vi "FP_Calibrate_reward.vi"() -> ()   [LabVIEW 2018]
uses:
  <vilib>/Instr/_visa.llb/VISA Flush IO Buffer Mask.ctl
  <vilib>/Utility/miscctls.llb/LVPointTypeDef.ctl
  Tracker.lvlib
panel:
  in  "O4 volume to dispense, µl":dbl=1.0 caption="Dispense, µl" min=0.0 max=10000.0 format="%#.3f"
  in  "O4 time to dispense, s":dbl=1.0 caption="Dispense, s" min=0.0 max=100.0 format="%.3g"
  in  "O4 Dispence, s":bool
  in  "O4 Dispence, µl":bool
  in  "O3 volume to dispense, µl":dbl=1.0 caption="Dispense, µl" min=0.0 max=10000.0 format="%#.3f"
  in  "O3 time to dispense, s":dbl=1.0 caption="Dispense, s" min=0.0 max=100.0 format="%.3g"
  in  "O3 Dispence, s":bool
  in  "O3 Dispence, µl":bool
  in  "O2 volume to dispense, µl":dbl=1.0 caption="Dispense, µl" min=0.0 max=10000.0 format="%#.3f"
  in  "O2 time to dispense, s":dbl=1.0 caption="Dispense, s" min=0.0 max=100.0 format="%.3g"
  in  "O2 Dispence, s":bool
  in  "O2 Dispence, µl":bool
  in  "O1 Dispence, µl":bool
  in  "O1 Dispence, s":bool
  in  "O1 time to dispense, s":dbl=1.0 caption="Dispense, s" min=0.0 max=100.0 format="%.3g"
  in  "O1 volume to dispense, µl":dbl=1.0 caption="Dispense, µl" min=0.0 max=10000.0 format="%#.3f"
  in  "O4 disp. time, s":dbl=1.0 min=0.0 max=100.0 format="%.3g"
  in  "O4 volume, µl":dbl=1.0 caption="Meas. volume, µl" min=0.0 max=10000.0 format="%#.3f"
  out "O4 speed, µl/s":dbl=1.0 caption="Speed, µl/s" format="%.3g"
  out "O4 act. disp. time, s":dbl=1.0 caption="Act. disp. time, s" format="%.3g"
  in  "O4 Disp. by time":bool
  in  "O3 disp. time, s":dbl=1.0 min=0.0 max=100.0 format="%.3g"
  in  "O3 volume, µl":dbl=1.0 caption="Meas. volume, µl" min=0.0 max=10000.0 format="%#.3f"
  out "O3 speed, µl/s":dbl=1.0 caption="Speed, µl/s" format="%.3g"
  out "O3 act. disp. time, s":dbl=1.0 caption="Act. disp. time, s" format="%.3g"
  in  "O3 Disp. by time":bool
  in  "O2 Disp. by time":bool
  in  "O2 disp. time, s":dbl=1.0 min=0.0 max=100.0 format="%.3g"
  in  "O2 volume, µl":dbl=1.0 caption="Meas. volume, µl" min=0.0 max=10000.0 format="%#.3f"
  out "O2 speed, µl/s":dbl=1.0 caption="Speed, µl/s" format="%.3g"
  out "O2 act. disp. time, s":dbl=1.0 caption="Act. disp. time, s" format="%.3g"
  out "O1 act. disp. time, s":dbl=1.0 caption="Act. disp. time, s" format="%.3g"
  out "O1 speed, µl/s":dbl=1.0 caption="Speed, µl/s" format="%.3g"
  in  "O1 volume, µl":dbl=1.0 caption="Meas. volume, µl" min=0.0 max=10000.0 format="%#.3f"
  in  "O1 Disp. by time":bool
  in  "O1 disp. time, s":dbl=1.0 min=0.0 max=100.0 format="%.3g"
  in  "Connect to HW":bool
  out "Ready":bool=TRUE
  out "HW info":string
  in  "Target FPS":i32=80 min=1 max=100 step=1
  in  "VISA resource":refnum<visa-resource-name>="Tracker"
  out "error out":errorcluster
  out "Sync capability":u8
  in  "error in":errorcluster
  # "O1"
  # "O2"
  # "O3"
  # "O4"
  # "Calibration"
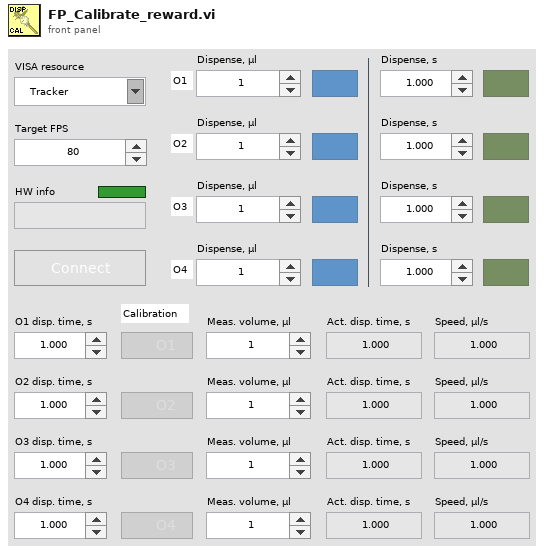
[diagram p1: front panel]
types:
  T1 = enum8{"Enabled", "Disabled", "Disabled and Grayed Out"}
  T2 = typedef "LVPointTypeDef.ctl" = cluster{"Horizontal":i16, "Vertical":i16}
  T3 = cluster{"SYNC configuration":u16, "IO 1 configuration":u16, "IO 2 configuration":u16, "IO 3 configuration":u16, "IO 4 configuration":u16, "Activate ext. RS-232":u16, "IO inversion config.":u16}
  T4 = typedef "VISA Flush IO Buffer Mask.ctl" = u16
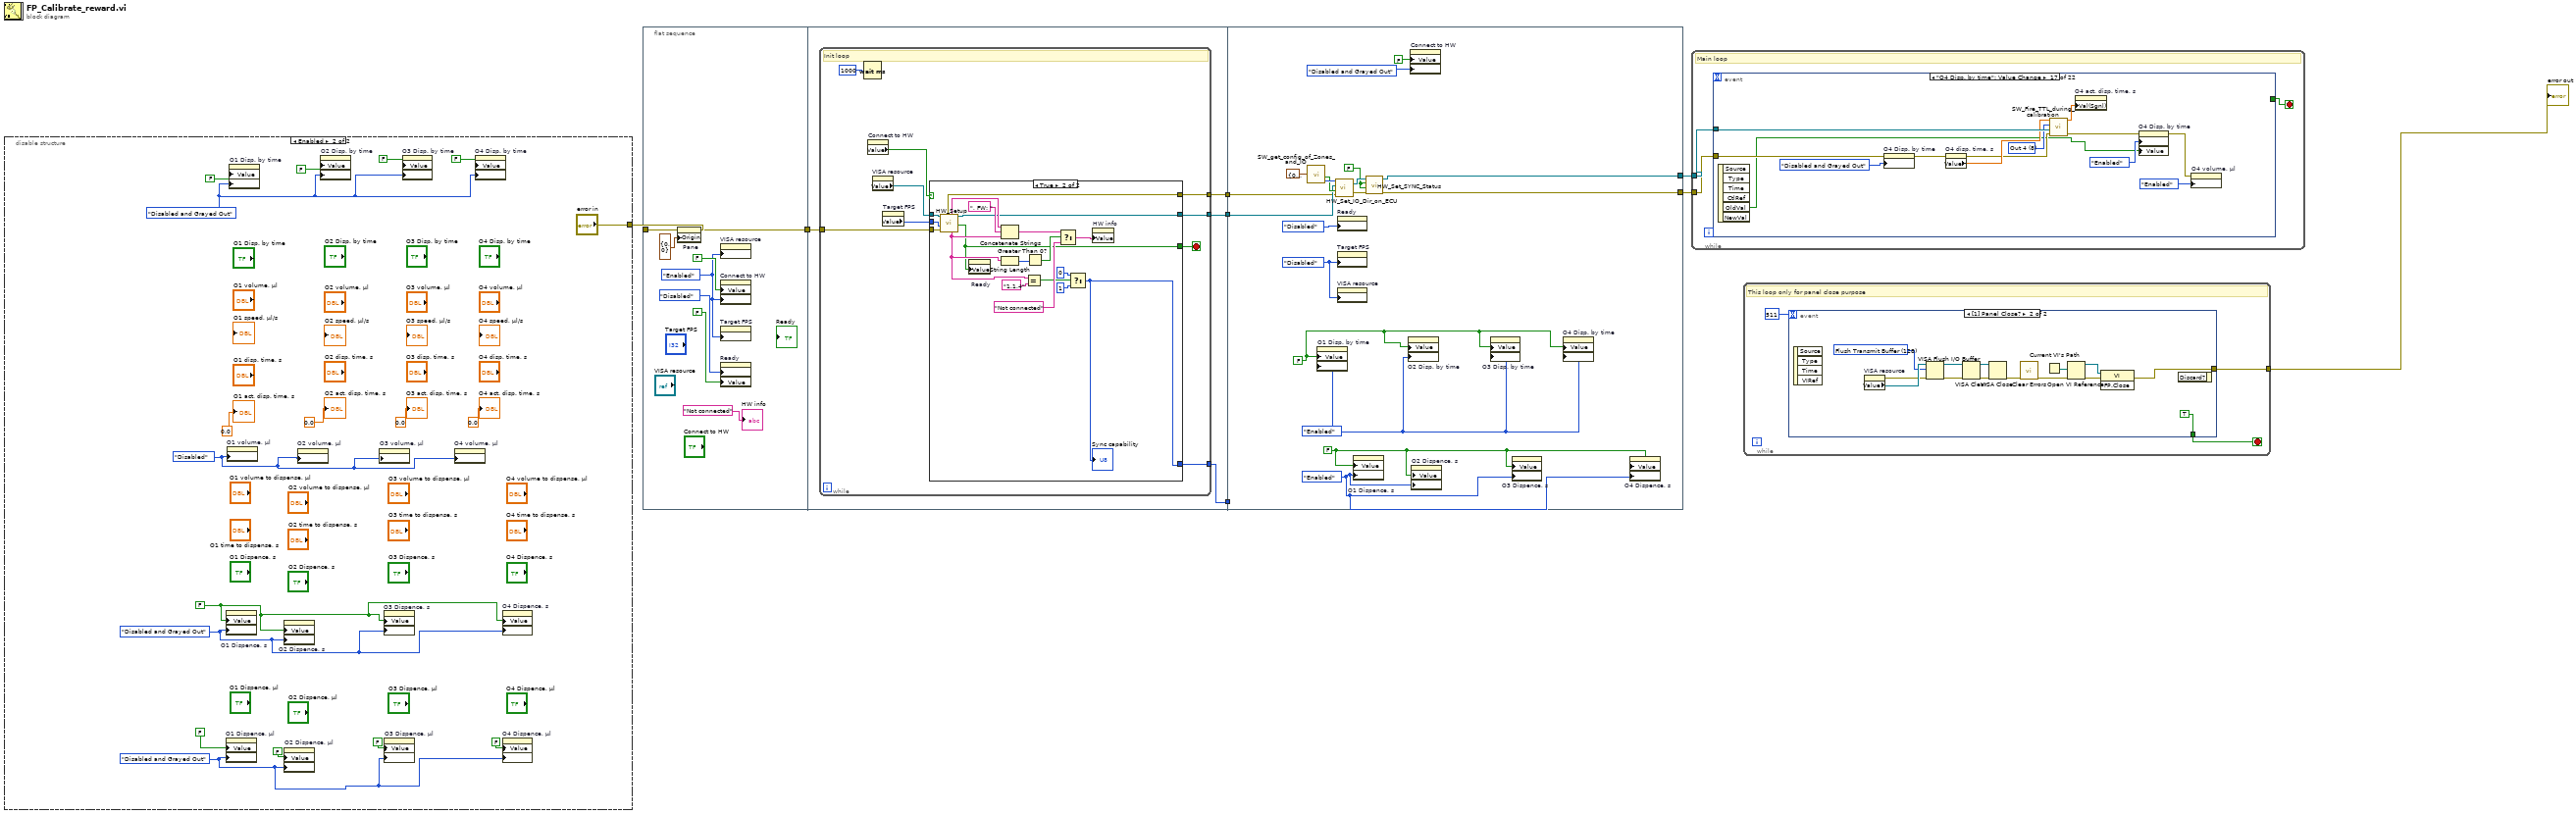
[diagram p0: block diagram]
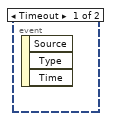
[diagram p2: hidden frame]
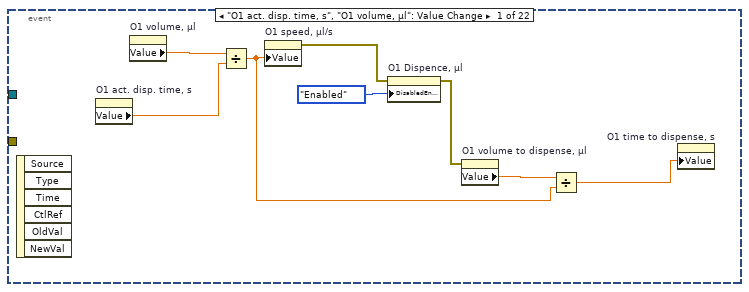
[diagram p3: hidden frame]
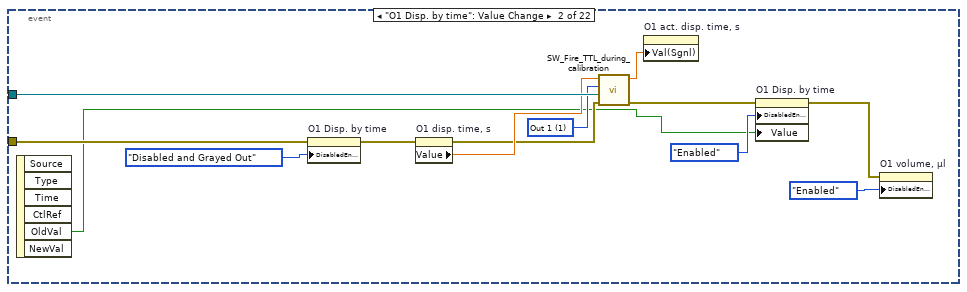
[diagram p4: hidden frame]
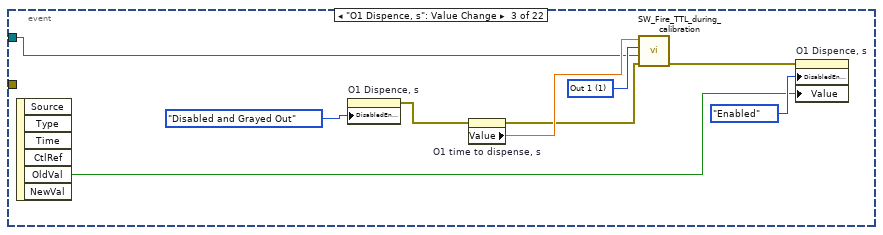
[diagram p5: hidden frame]
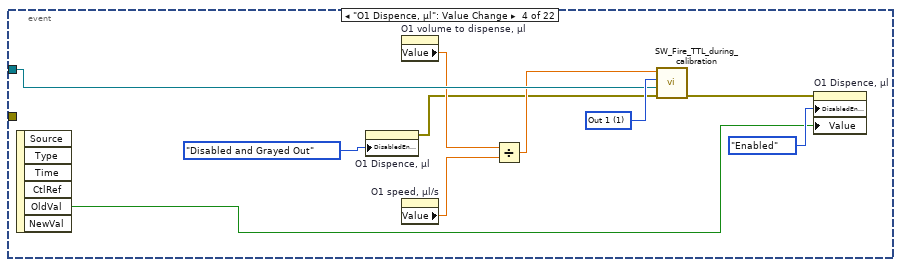
[diagram p6: hidden frame]
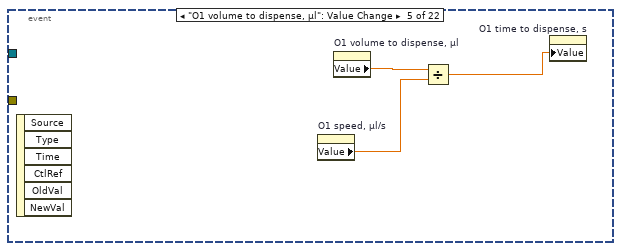
[diagram p7: hidden frame]
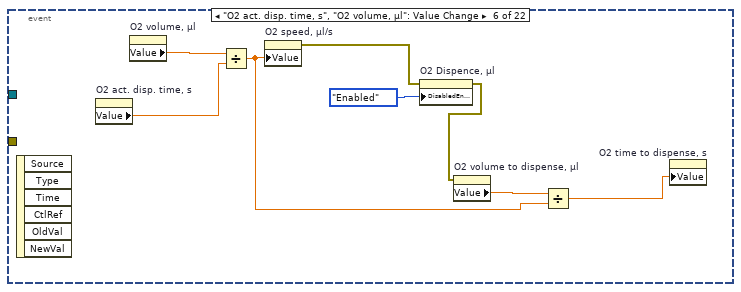
[diagram p8: hidden frame]
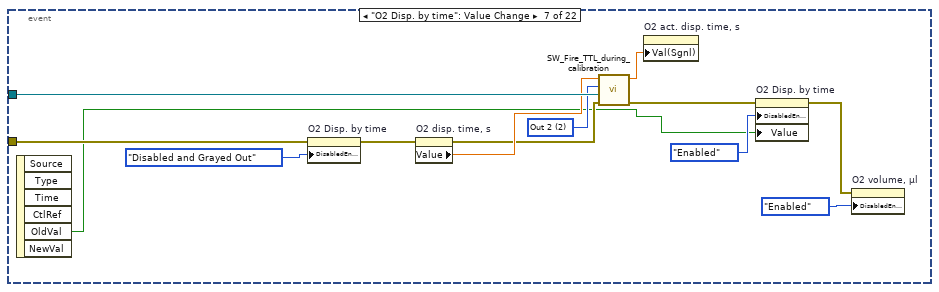
[diagram p9: hidden frame]
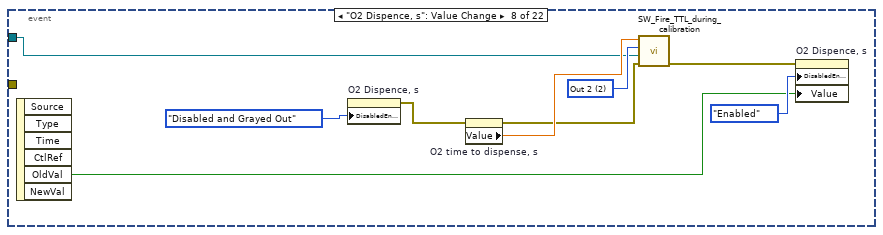
[diagram p10: hidden frame]
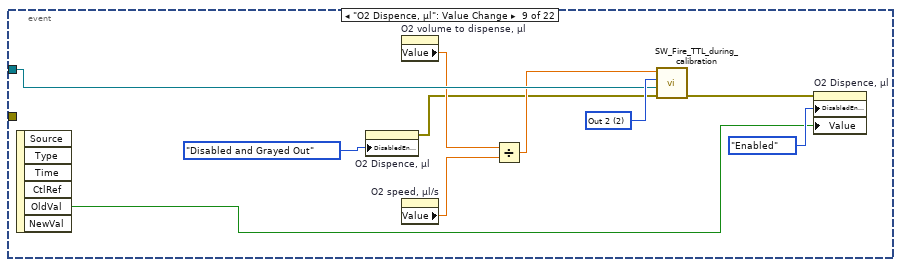
[diagram p11: hidden frame]
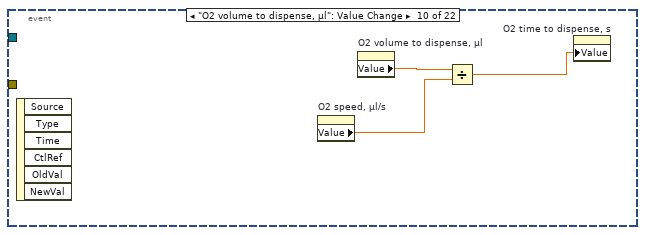
[diagram p12: hidden frame]
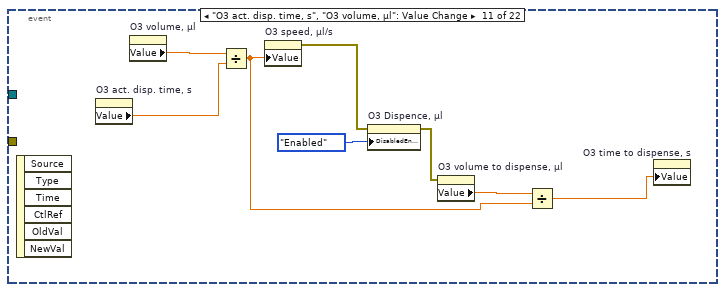
[diagram p13: hidden frame]
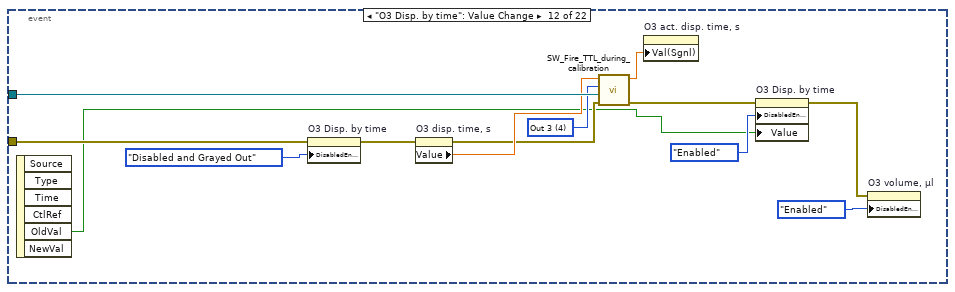
[diagram p14: hidden frame]
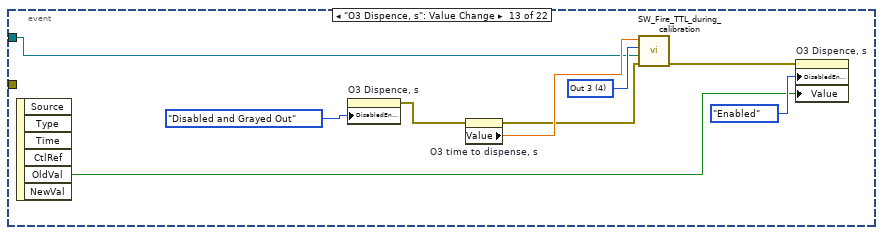
[diagram p15: hidden frame]
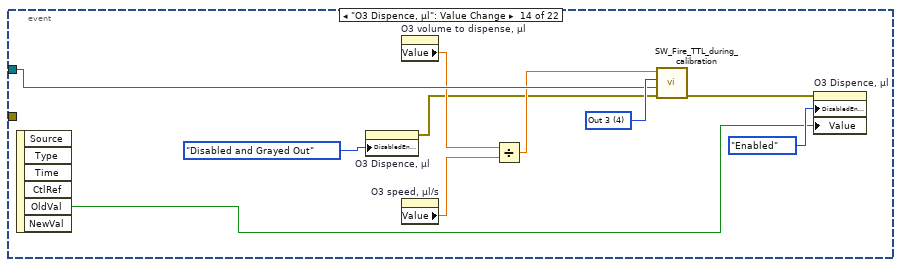
[diagram p16: hidden frame]
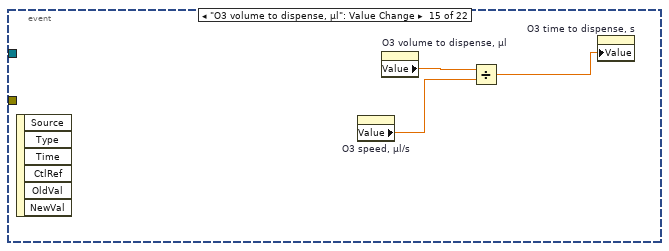
[diagram p17: hidden frame]
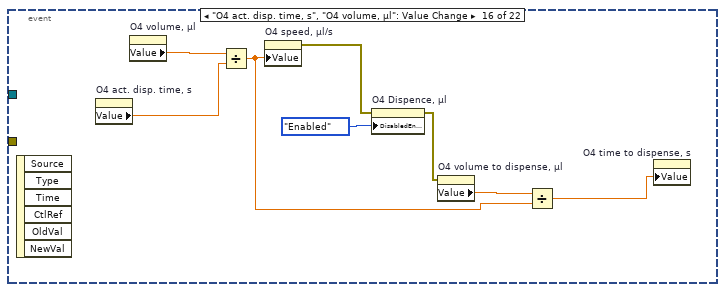
[diagram p18: hidden frame]
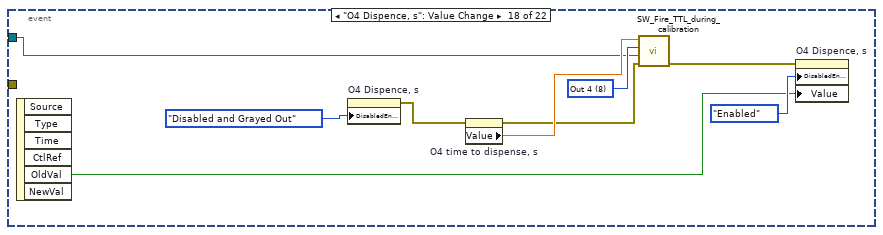
[diagram p19: hidden frame]
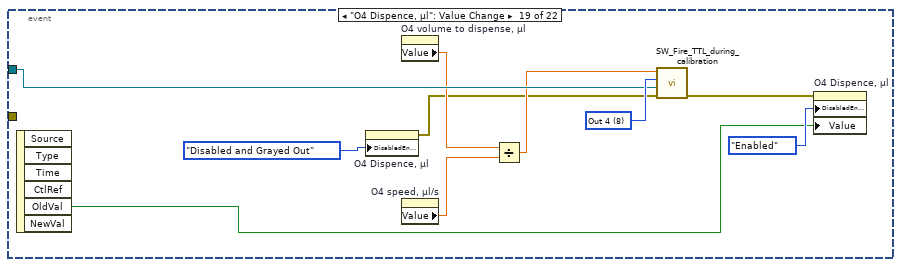
[diagram p20: hidden frame]
diagram:
  n1 = disable-structure shown="Enabled" {
    disable-tunnel: [_ "error in"] -> w4
    frame Disabled {
    }
    frame Enabled {
      w9 = T1."Disabled" ("Disabled")
      w11 = T1."Disabled and Grayed Out" ("Disabled")
      w12 = T1."Disabled and Grayed Out" ("Disabled")
      w13 = T1."Disabled and Grayed Out" ("Disabled")
      w10 = FALSE ("O1 Dispence, s")
      n2 = property on="O1 Dispence, s" class="Bool (strict)"("Value"=w10, "DisabledEnum"=w12) -> ()  [unwired: 2 in, 2 out]
      n3 = property on="O1 Dispence, µl" class="Bool (strict)"("Value"=FALSE ("O1 Dispence, µl"), "DisabledEnum"=w11) -> ()  [unwired: 2 in, 2 out]
      n4 = property on="O1 volume, µl" class="DigNum (strict)"("DisabledEnum"=w9) -> ()  [unwired: 2 in, 2 out]
      n5 = property on="O1 Disp. by time" class="Bool (strict)"("Value"=FALSE ("O1 Disp. by time"), "DisabledEnum"=w13) -> ()  [unwired: 2 in, 2 out]
      n6 = property on="O2 Dispence, s" class="Bool (strict)"("Value"=w10, "DisabledEnum"=w12) -> ()  [unwired: 2 in, 2 out]
      n7 = property on="O2 Dispence, µl" class="Bool (strict)"("Value"=FALSE ("O1 Dispence, µl"), "DisabledEnum"=w11) -> ()  [unwired: 2 in, 2 out]
      n8 = property on="O2 volume, µl" class="DigNum (strict)"("DisabledEnum"=w9) -> ()  [unwired: 2 in, 2 out]
      n9 = property on="O2 Disp. by time" class="Bool (strict)"("Value"=FALSE ("O1 Disp. by time"), "DisabledEnum"=w13) -> ()  [unwired: 2 in, 2 out]
      n10 = property on="O3 volume, µl" class="DigNum (strict)"("DisabledEnum"=w9) -> ()  [unwired: 2 in, 2 out]
      n11 = property on="O3 Dispence, s" class="Bool (strict)"("Value"=w10, "DisabledEnum"=w12) -> ()  [unwired: 2 in, 2 out]
      n12 = property on="O3 Dispence, µl" class="Bool (strict)"("Value"=FALSE ("O1 Dispence, µl"), "DisabledEnum"=w11) -> ()  [unwired: 2 in, 2 out]
      n13 = property on="O3 Disp. by time" class="Bool (strict)"("Value"=FALSE ("O1 Disp. by time"), "DisabledEnum"=w13) -> ()  [unwired: 2 in, 2 out]
      n14 = property on="O4 volume, µl" class="DigNum (strict)"("DisabledEnum"=w9) -> ()  [unwired: 2 in, 2 out]
      n15 = property on="O4 Disp. by time" class="Bool (strict)"("Value"=FALSE ("O1 Disp. by time"), "DisabledEnum"=w13) -> ()  [unwired: 2 in, 2 out]
      n16 = property on="O4 Dispence, s" class="Bool (strict)"("Value"=w10, "DisabledEnum"=w12) -> ()  [unwired: 2 in, 2 out]
      n17 = property on="O4 Dispence, µl" class="Bool (strict)"("Value"=FALSE ("O1 Dispence, µl"), "DisabledEnum"=w11) -> ()  [unwired: 2 in, 2 out]
      "O1 act. disp. time, s" <- 0.0 ("Act. disp. time, s")
      "O2 act. disp. time, s" <- 0.0 ("Act. disp. time, s")
      "O3 act. disp. time, s" <- 0.0 ("Act. disp. time, s")
      "O4 act. disp. time, s" <- 0.0 ("Act. disp. time, s")
    }
  }
  n18 = flat-sequence {
    tunnel: [w33] -> w8
    tunnel: w4 -> [w27]
    tunnel: w8 -> [w37]
    tunnel: [w38] -> w7
    tunnel: [w36] -> w6
    tunnel: [w35] -> w5
    tunnel: w7 -> [w79]
    tunnel: w6 -> [_]
    tunnel: w5 -> [w82]
    tunnel: [w76] -> w3
    tunnel: [w75] -> w2
    frame #0 {
      w28 = T1."Enabled" ("Disabled")
      n19 = property on="Pane" class="Pane"(error in=w27, "Origin"=T2 {"Horizontal"=0, "Vertical"=0}) -> (error out=w33:errorcluster)  [unwired: 1 in, 1 out]
      n20 = property on="VISA resource" class="VISAName"("DisabledEnum"=w28) -> ()  [unwired: 2 in, 2 out]
      n21 = property on="Connect to HW" class="Bool (strict)"("Value"=FALSE ("Connect to HW"), "DisabledEnum"=w28) -> ()  [unwired: 2 in, 2 out]
      n22 = property on="Target FPS" class="DigNum (strict)"("DisabledEnum"=w28) -> ()  [unwired: 2 in, 2 out]
      n23 = property on="Ready" class="Bool (strict)"("DisabledEnum"=T1."Disabled" ("Disabled"), "Value"=FALSE ("Ready")) -> ()  [unwired: 2 in, 2 out]
      "HW info" <- "Not connected" ("HW info")
    }
    frame #1 {
      n24 = while {
        tunnel: [w47] -> w38
        tunnel: w37 -> [w46]
        tunnel: [w40] -> w36
        tunnel: [w39] -> w35
        stop <- w44 stop-if-true
        # "Init loop"
        n25 = Wait (ms)(milliseconds to wait=u32 1000) -> ()  [unwired: 1 out]
        n26 = property on="Connect to HW" class="Bool (strict)"() -> ("Value"=w43:bool)  [unwired: 2 in, 2 out]
        n27 = property on="VISA resource" class="VISAName"() -> ("Value"=w42:refnum<visa-resource-name>)  [unwired: 2 in, 2 out]
        n28 = property on="Target FPS" class="DigNum (strict)"() -> ("Value"=w41:i32)  [unwired: 2 in, 2 out]
        n29 = case shown="True" w43 {
          tunnel: [w51 w70] -> w47
          tunnel: w46 -> [w51 w69]
          tunnel: [FALSE ("Instrument OK?") w57] -> w44
          tunnel: w42 -> [w48 w56]
          tunnel: w41 -> [_ w55]
          tunnel: [u8 0 ("f") w53] -> w40
          tunnel: [w48 w52] -> w39
          frame False {
          }
          frame True {
            n30 = call "HW_Setup.vi"("error in"=w69, "Traget FPS"=w55, "VISA resource name in"=w56) -> ("Instrument OK?"=w57:bool, "VISA resource name out"=w52:refnum<visa-resource-name>, "Version information"=w58:string, "Sensor board size"=w59:string, "error out"=w70:errorcluster)  [unwired: 1 in, 3 out]
            n31 = property on="Ready" class="Bool (strict)"("Value"=w57) -> ()  [unwired: 2 in, 2 out]
            n32 = Concatenate Strings(w59, ", FW: " ("string"), w58) -> (w65:string)
            n33 = String Length(string=w58) -> (length=w67:i32)
            n34 = Equal?(x=w58, y="1.1.4") -> (x = y?=w62:bool)
            n35 = Greater Than 0?(x=w67) -> (x > 0?=w66:bool)
            n36 = Select(t=w65, s=w66, f="Not connected") -> (s? t:f=w54:string)
            n37 = Select(t=u8 0, s=w62, f=u8 1) -> (s? t:f=w53:u8)
            "Sync capability" <- w53
            n38 = property on="HW info" class="Str"("Value"=w54) -> ()  [unwired: 2 in, 2 out]
          }
        }
      }
    }
    frame #2 {
      w72 = T1."Enabled" ("Disabled")
      w73 = FALSE ("O1 Dispence, s")
      w74 = T1."Enabled" ("Disabled")
      w71 = FALSE ("O1 Disp. by time")
      w78 = FALSE
      w88 = T1."Disabled" ("Disabled")
      n39 = call "SW_get_config_of_Zones_and_IO.vi"("Sync parameters cluster input"=T3 {"SYNC configuration"=0, "IO 1 configuration"=1, "IO 2 configuration"=1, "IO 3 configuration"=1, "IO 4 configuration"=1, "Activate ext. RS-232"=0, "IO inversion config."=0} ("IO config cluster for calibration case")) -> ("Ports IO config (OUT is FALSE)"=w83:bool[], "IO inversion config."=w84:u16)  [unwired: 2 out]
      n40 = property on="O1 Disp. by time" class="Bool (strict)"("Value"=w71, "DisabledEnum"=w74) -> ()  [unwired: 2 in, 2 out]
      n41 = call "HW_Set_IO_Dir_on_ECU.vi"("Error In"=w79, "IO ports config"=w83, "VISA resource name"=w82, "IO inversion config."=w84) -> ("error out"=w80:errorcluster, "VISA resource name out"=w81:refnum<visa-resource-name>)
      n42 = property on="Ready" class="Bool (strict)"("DisabledEnum"=T1."Disabled" ("Disabled")) -> ()  [unwired: 2 in, 2 out]
      n43 = property on="Target FPS" class="DigNum (strict)"("DisabledEnum"=w88) -> ()  [unwired: 2 in, 2 out]
      n44 = property on="VISA resource" class="VISAName"("DisabledEnum"=w88) -> ()  [unwired: 2 in, 2 out]
      n45 = property on="O1 Dispence, s" class="Bool (strict)"("Value"=w73, "DisabledEnum"=w72) -> ()  [unwired: 2 in, 2 out]
      n46 = call "HW_Set_SYNC_Status.vi"("error in (no error)"=w80, "SYNC 2"=w78, "SYNC 1"=w78, "VISA Resource name IN"=w81) -> ("error out"=w76:errorcluster, "VISA resource name out"=w75:refnum<visa-resource-name>)  [unwired: 6 in]
      n47 = property on="O2 Disp. by time" class="Bool (strict)"("Value"=w71, "DisabledEnum"=w74) -> ()  [unwired: 2 in, 2 out]
      n48 = property on="Connect to HW" class="Bool (strict)"("Value"=FALSE ("Connect to HW"), "DisabledEnum"=T1."Disabled and Grayed Out" ("Disabled")) -> ()  [unwired: 2 in, 2 out]
      n49 = property on="O2 Dispence, s" class="Bool (strict)"("Value"=w73, "DisabledEnum"=w72) -> ()  [unwired: 2 in, 2 out]
      n50 = property on="O3 Disp. by time" class="Bool (strict)"("Value"=w71, "DisabledEnum"=w74) -> ()  [unwired: 2 in, 2 out]
      n51 = property on="O3 Dispence, s" class="Bool (strict)"("Value"=w73, "DisabledEnum"=w72) -> ()  [unwired: 2 in, 2 out]
      n52 = property on="O4 Disp. by time" class="Bool (strict)"("Value"=w71, "DisabledEnum"=w74) -> ()  [unwired: 2 in, 2 out]
      n53 = property on="O4 Dispence, s" class="Bool (strict)"("Value"=w73, "DisabledEnum"=w72) -> ()  [unwired: 2 in, 2 out]
    }
  }
  n54 = while {
    tunnel: w3 -> [w89]
    tunnel: w2 -> [w90]
    stop <- w91 stop-if-true
    # "Main loop"
    n55 = event shown="[16] \"O4 Disp. by time\": Value Change" {
      selector: _ -> [_ _ _ _ _ _ _ _ _ _ _ _ _ _ _ _ _ _ _ _ _ _]
      dyn-events: _ -> [_ _ _ _ _ _ _ _ _ _ _ _ _ _ _ _ _ _ _ _ _ _]
      timeout: _ -> [_ _ _ _ _ _ _ _ _ _ _ _ _ _ _ _ _ _ _ _ _ _]
      tunnel: [_ _ _ _ _ _ _ _ _ _ _ _ _ _ _ _ _ _ _ _ TRUE FALSE] -> w91
      tunnel: w90 -> [_ w112 w114 w127 _ _ w155 w157 w170 _ _ w198 w200 w213 _ _ w241 w243 w256 _ _ _]
      tunnel: w89 -> [_ w107 _ _ _ _ w150 _ _ _ _ w193 _ _ _ _ w236 _ _ _ _ _]
      event "O1 act. disp. time, s", "O1 volume, µl": Value Change {
        n56 = event-data() -> ()  [unwired: 1 in, 6 out]
        n57 = property on="O1 act. disp. time, s" class="DigNum (strict)"() -> ("Value"=w98:dbl)  [unwired: 2 in, 2 out]
        n58 = property on="O1 volume, µl" class="DigNum (strict)"() -> ("Value"=w99:dbl)  [unwired: 2 in, 2 out]
        n59 = Divide(x=w99, y=w98) -> (x/y=w93:dbl)
        n60 = property on="O1 speed, µl/s" class="DigNum (strict)"("Value"=w93) -> (error out=w96:errorcluster)  [unwired: 2 in, 1 out]
        n61 = property on="O1 Dispence, µl" class="Bool (strict)"(error in=w96, "DisabledEnum"=T1."Enabled" ("Disabled")) -> (error out=w92:errorcluster)  [unwired: 1 in, 1 out]
        n62 = property on="O1 volume to dispense, µl" class="DigNum (strict)"(error in=w92) -> ("Value"=w95:dbl)  [unwired: 1 in, 2 out]
        n63 = Divide(x=w95, y=w93) -> (x/y=w94:dbl)
        n64 = property on="O1 time to dispense, s" class="DigNum (strict)"("Value"=w94) -> ()  [unwired: 2 in, 2 out]
      }
      event "O1 Disp. by time": Value Change {
        w109 = u16 1 items=["Out 1"=1, "Out 2"=2, "Out 3"=4, "Out 4"=8] ("Port to fire")
        n65 = event-data() -> ("OldVal"=w102:bool)  [unwired: 1 in, 5 out]
        n66 = property on="O1 Disp. by time" class="Bool (strict)"(error in=w107, "DisabledEnum"=T1."Disabled and Grayed Out" ("Disabled")) -> (error out=w108:errorcluster)  [unwired: 1 in, 1 out]
        n67 = property on="O1 disp. time, s" class="DigNum (strict)"(error in=w108) -> (error out=w106:errorcluster, "Value"=w111:dbl)  [unwired: 1 in, 1 out]
        n68 = call "SW_Fire_TTL_during_calibration.vi"("error in (no error)"=w106, "VISA resource in"=w112, "Port to fire"=w109, "TTL pulse length, s"=w111) -> ("error out"=w103:errorcluster, "Time spent to process command, s"=w110:dbl)  [unwired: 5 in, 1 out]
        n69 = property on="O1 act. disp. time, s" class="DigNum (strict)"("Val(Sgnl)"=w110) -> ()  [unwired: 2 in, 2 out]
        n70 = property on="O1 Disp. by time" class="Bool (strict)"(error in=w103, "DisabledEnum"=T1."Enabled" ("Disabled"), "Value"=w102) -> (error out=w100:errorcluster)  [unwired: 1 in, 1 out]
        n71 = property on="O1 volume, µl" class="DigNum (strict)"(error in=w100, "DisabledEnum"=T1."Enabled" ("Disabled")) -> ()  [unwired: 1 in, 2 out]
      }
      event "O1 Dispence, s": Value Change {
        w120 = u16 1 items=["Out 1"=1, "Out 2"=2, "Out 3"=4, "Out 4"=8] ("Port to fire")
        n72 = event-data() -> ("OldVal"=w113:bool)  [unwired: 1 in, 5 out]
        n73 = property on="O1 Dispence, s" class="Bool (strict)"("DisabledEnum"=T1."Disabled and Grayed Out" ("Disabled")) -> (error out=w119:errorcluster)  [unwired: 2 in, 1 out]
        n74 = property on="O1 time to dispense, s" class="DigNum (strict)"(error in=w119) -> (error out=w118:errorcluster, "Value"=w121:dbl)  [unwired: 1 in, 1 out]
        n75 = call "SW_Fire_TTL_during_calibration.vi"("error in (no error)"=w118, "VISA resource in"=w114, "Port to fire"=w120, "TTL pulse length, s"=w121) -> ("error out"=w115:errorcluster)  [unwired: 5 in, 2 out]
        n76 = property on="O1 Dispence, s" class="Bool (strict)"(error in=w115, "DisabledEnum"=T1."Enabled" ("Disabled"), "Value"=w113) -> ()  [unwired: 1 in, 2 out]
      }
      event "O1 Dispence, µl": Value Change {
        w131 = u16 1 items=["Out 1"=1, "Out 2"=2, "Out 3"=4, "Out 4"=8] ("Port to fire")
        n77 = event-data() -> ("OldVal"=w123:bool)  [unwired: 1 in, 5 out]
        n78 = property on="O1 Dispence, µl" class="Bool (strict)"("DisabledEnum"=T1."Disabled and Grayed Out" ("Disabled")) -> (error out=w122:errorcluster)  [unwired: 2 in, 1 out]
        n79 = property on="O1 volume to dispense, µl" class="DigNum (strict)"() -> ("Value"=w125:dbl)  [unwired: 2 in, 2 out]
        n80 = property on="O1 speed, µl/s" class="DigNum (strict)"() -> ("Value"=w126:dbl)  [unwired: 2 in, 2 out]
        n81 = Divide(x=w125, y=w126) -> (x/y=w124:dbl)
        n82 = call "SW_Fire_TTL_during_calibration.vi"("error in (no error)"=w122, "VISA resource in"=w127, "Port to fire"=w131, "TTL pulse length, s"=w124) -> ("error out"=w128:errorcluster)  [unwired: 5 in, 2 out]
        n83 = property on="O1 Dispence, µl" class="Bool (strict)"(error in=w128, "DisabledEnum"=T1."Enabled" ("Disabled"), "Value"=w123) -> ()  [unwired: 1 in, 2 out]
      }
      event "O1 volume to dispense, µl": Value Change {
        n84 = event-data() -> ()  [unwired: 1 in, 6 out]
        n85 = property on="O1 speed, µl/s" class="DigNum (strict)"() -> ("Value"=w132:dbl)  [unwired: 2 in, 2 out]
        n86 = property on="O1 volume to dispense, µl" class="DigNum (strict)"() -> ("Value"=w134:dbl)  [unwired: 2 in, 2 out]
        n87 = Divide(x=w134, y=w132) -> (x/y=w133:dbl)
        n88 = property on="O1 time to dispense, s" class="DigNum (strict)"("Value"=w133) -> ()  [unwired: 2 in, 2 out]
      }
      event "O2 act. disp. time, s", "O2 volume, µl": Value Change {
        n89 = event-data() -> ()  [unwired: 1 in, 6 out]
        n90 = property on="O2 act. disp. time, s" class="DigNum (strict)"() -> ("Value"=w141:dbl)  [unwired: 2 in, 2 out]
        n91 = property on="O2 volume, µl" class="DigNum (strict)"() -> ("Value"=w142:dbl)  [unwired: 2 in, 2 out]
        n92 = Divide(x=w142, y=w141) -> (x/y=w135:dbl)
        n93 = property on="O2 speed, µl/s" class="DigNum (strict)"("Value"=w135) -> (error out=w139:errorcluster)  [unwired: 2 in, 1 out]
        n94 = property on="O2 Dispence, µl" class="Bool (strict)"(error in=w139, "DisabledEnum"=T1."Enabled" ("Disabled")) -> (error out=w136:errorcluster)  [unwired: 1 in, 1 out]
        n95 = property on="O2 volume to dispense, µl" class="DigNum (strict)"(error in=w136) -> ("Value"=w138:dbl)  [unwired: 1 in, 2 out]
        n96 = Divide(x=w138, y=w135) -> (x/y=w137:dbl)
        n97 = property on="O2 time to dispense, s" class="DigNum (strict)"("Value"=w137) -> ()  [unwired: 2 in, 2 out]
      }
      event "O2 Disp. by time": Value Change {
        w152 = u16 2 items=["Out 1"=1, "Out 2"=2, "Out 3"=4, "Out 4"=8] ("Port to fire")
        n98 = event-data() -> ("OldVal"=w145:bool)  [unwired: 1 in, 5 out]
        n99 = property on="O2 Disp. by time" class="Bool (strict)"(error in=w150, "DisabledEnum"=T1."Disabled and Grayed Out" ("Disabled")) -> (error out=w151:errorcluster)  [unwired: 1 in, 1 out]
        n100 = property on="O2 disp. time, s" class="DigNum (strict)"(error in=w151) -> (error out=w149:errorcluster, "Value"=w154:dbl)  [unwired: 1 in, 1 out]
        n101 = call "SW_Fire_TTL_during_calibration.vi"("error in (no error)"=w149, "VISA resource in"=w155, "Port to fire"=w152, "TTL pulse length, s"=w154) -> ("error out"=w146:errorcluster, "Time spent to process command, s"=w153:dbl)  [unwired: 5 in, 1 out]
        n102 = property on="O2 act. disp. time, s" class="DigNum (strict)"("Val(Sgnl)"=w153) -> ()  [unwired: 2 in, 2 out]
        n103 = property on="O2 Disp. by time" class="Bool (strict)"(error in=w146, "DisabledEnum"=T1."Enabled" ("Disabled"), "Value"=w145) -> (error out=w143:errorcluster)  [unwired: 1 in, 1 out]
        n104 = property on="O2 volume, µl" class="DigNum (strict)"(error in=w143, "DisabledEnum"=T1."Enabled" ("Disabled")) -> ()  [unwired: 1 in, 2 out]
      }
      event "O2 Dispence, s": Value Change {
        w163 = u16 2 items=["Out 1"=1, "Out 2"=2, "Out 3"=4, "Out 4"=8] ("Port to fire")
        n105 = event-data() -> ("OldVal"=w156:bool)  [unwired: 1 in, 5 out]
        n106 = property on="O2 Dispence, s" class="Bool (strict)"("DisabledEnum"=T1."Disabled and Grayed Out" ("Disabled")) -> (error out=w162:errorcluster)  [unwired: 2 in, 1 out]
        n107 = property on="O2 time to dispense, s" class="DigNum (strict)"(error in=w162) -> (error out=w161:errorcluster, "Value"=w164:dbl)  [unwired: 1 in, 1 out]
        n108 = call "SW_Fire_TTL_during_calibration.vi"("error in (no error)"=w161, "VISA resource in"=w157, "Port to fire"=w163, "TTL pulse length, s"=w164) -> ("error out"=w158:errorcluster)  [unwired: 5 in, 2 out]
        n109 = property on="O2 Dispence, s" class="Bool (strict)"(error in=w158, "DisabledEnum"=T1."Enabled" ("Disabled"), "Value"=w156) -> ()  [unwired: 1 in, 2 out]
      }
      event "O2 Dispence, µl": Value Change {
        w174 = u16 2 items=["Out 1"=1, "Out 2"=2, "Out 3"=4, "Out 4"=8] ("Port to fire")
        n110 = event-data() -> ("OldVal"=w166:bool)  [unwired: 1 in, 5 out]
        n111 = property on="O2 Dispence, µl" class="Bool (strict)"("DisabledEnum"=T1."Disabled and Grayed Out" ("Disabled")) -> (error out=w165:errorcluster)  [unwired: 2 in, 1 out]
        n112 = property on="O2 volume to dispense, µl" class="DigNum (strict)"() -> ("Value"=w168:dbl)  [unwired: 2 in, 2 out]
        n113 = property on="O2 speed, µl/s" class="DigNum (strict)"() -> ("Value"=w169:dbl)  [unwired: 2 in, 2 out]
        n114 = Divide(x=w168, y=w169) -> (x/y=w167:dbl)
        n115 = call "SW_Fire_TTL_during_calibration.vi"("error in (no error)"=w165, "VISA resource in"=w170, "Port to fire"=w174, "TTL pulse length, s"=w167) -> ("error out"=w171:errorcluster)  [unwired: 5 in, 2 out]
        n116 = property on="O2 Dispence, µl" class="Bool (strict)"(error in=w171, "DisabledEnum"=T1."Enabled" ("Disabled"), "Value"=w166) -> ()  [unwired: 1 in, 2 out]
      }
      event "O2 volume to dispense, µl": Value Change {
        n117 = event-data() -> ()  [unwired: 1 in, 6 out]
        n118 = property on="O2 speed, µl/s" class="DigNum (strict)"() -> ("Value"=w175:dbl)  [unwired: 2 in, 2 out]
        n119 = property on="O2 volume to dispense, µl" class="DigNum (strict)"() -> ("Value"=w177:dbl)  [unwired: 2 in, 2 out]
        n120 = Divide(x=w177, y=w175) -> (x/y=w176:dbl)
        n121 = property on="O2 time to dispense, s" class="DigNum (strict)"("Value"=w176) -> ()  [unwired: 2 in, 2 out]
      }
      event "O3 act. disp. time, s", "O3 volume, µl": Value Change {
        n122 = event-data() -> ()  [unwired: 1 in, 6 out]
        n123 = property on="O3 act. disp. time, s" class="DigNum (strict)"() -> ("Value"=w184:dbl)  [unwired: 2 in, 2 out]
        n124 = property on="O3 volume, µl" class="DigNum (strict)"() -> ("Value"=w185:dbl)  [unwired: 2 in, 2 out]
        n125 = Divide(x=w185, y=w184) -> (x/y=w179:dbl)
        n126 = property on="O3 speed, µl/s" class="DigNum (strict)"("Value"=w179) -> (error out=w182:errorcluster)  [unwired: 2 in, 1 out]
        n127 = property on="O3 Dispence, µl" class="Bool (strict)"(error in=w182, "DisabledEnum"=T1."Enabled" ("Disabled")) -> (error out=w178:errorcluster)  [unwired: 1 in, 1 out]
        n128 = property on="O3 volume to dispense, µl" class="DigNum (strict)"(error in=w178) -> ("Value"=w181:dbl)  [unwired: 1 in, 2 out]
        n129 = Divide(x=w181, y=w179) -> (x/y=w180:dbl)
        n130 = property on="O3 time to dispense, s" class="DigNum (strict)"("Value"=w180) -> ()  [unwired: 2 in, 2 out]
      }
      event "O3 Disp. by time": Value Change {
        w195 = u16 4 items=["Out 1"=1, "Out 2"=2, "Out 3"=4, "Out 4"=8] ("Port to fire")
        n131 = event-data() -> ("OldVal"=w188:bool)  [unwired: 1 in, 5 out]
        n132 = property on="O3 Disp. by time" class="Bool (strict)"(error in=w193, "DisabledEnum"=T1."Disabled and Grayed Out" ("Disabled")) -> (error out=w194:errorcluster)  [unwired: 1 in, 1 out]
        n133 = property on="O3 disp. time, s" class="DigNum (strict)"(error in=w194) -> (error out=w192:errorcluster, "Value"=w197:dbl)  [unwired: 1 in, 1 out]
        n134 = call "SW_Fire_TTL_during_calibration.vi"("error in (no error)"=w192, "VISA resource in"=w198, "Port to fire"=w195, "TTL pulse length, s"=w197) -> ("error out"=w189:errorcluster, "Time spent to process command, s"=w196:dbl)  [unwired: 5 in, 1 out]
        n135 = property on="O3 act. disp. time, s" class="DigNum (strict)"("Val(Sgnl)"=w196) -> ()  [unwired: 2 in, 2 out]
        n136 = property on="O3 Disp. by time" class="Bool (strict)"(error in=w189, "DisabledEnum"=T1."Enabled" ("Disabled"), "Value"=w188) -> (error out=w186:errorcluster)  [unwired: 1 in, 1 out]
        n137 = property on="O3 volume, µl" class="DigNum (strict)"(error in=w186, "DisabledEnum"=T1."Enabled" ("Disabled")) -> ()  [unwired: 1 in, 2 out]
      }
      event "O3 Dispence, s": Value Change {
        w206 = u16 4 items=["Out 1"=1, "Out 2"=2, "Out 3"=4, "Out 4"=8] ("Port to fire")
        n138 = event-data() -> ("OldVal"=w199:bool)  [unwired: 1 in, 5 out]
        n139 = property on="O3 Dispence, s" class="Bool (strict)"("DisabledEnum"=T1."Disabled and Grayed Out" ("Disabled")) -> (error out=w205:errorcluster)  [unwired: 2 in, 1 out]
        n140 = property on="O3 time to dispense, s" class="DigNum (strict)"(error in=w205) -> (error out=w204:errorcluster, "Value"=w207:dbl)  [unwired: 1 in, 1 out]
        n141 = call "SW_Fire_TTL_during_calibration.vi"("error in (no error)"=w204, "VISA resource in"=w200, "Port to fire"=w206, "TTL pulse length, s"=w207) -> ("error out"=w201:errorcluster)  [unwired: 5 in, 2 out]
        n142 = property on="O3 Dispence, s" class="Bool (strict)"(error in=w201, "DisabledEnum"=T1."Enabled" ("Disabled"), "Value"=w199) -> ()  [unwired: 1 in, 2 out]
      }
      event "O3 Dispence, µl": Value Change {
        w217 = u16 4 items=["Out 1"=1, "Out 2"=2, "Out 3"=4, "Out 4"=8] ("Port to fire")
        n143 = event-data() -> ("OldVal"=w209:bool)  [unwired: 1 in, 5 out]
        n144 = property on="O3 Dispence, µl" class="Bool (strict)"("DisabledEnum"=T1."Disabled and Grayed Out" ("Disabled")) -> (error out=w208:errorcluster)  [unwired: 2 in, 1 out]
        n145 = property on="O3 volume to dispense, µl" class="DigNum (strict)"() -> ("Value"=w211:dbl)  [unwired: 2 in, 2 out]
        n146 = property on="O3 speed, µl/s" class="DigNum (strict)"() -> ("Value"=w212:dbl)  [unwired: 2 in, 2 out]
        n147 = Divide(x=w211, y=w212) -> (x/y=w210:dbl)
        n148 = call "SW_Fire_TTL_during_calibration.vi"("error in (no error)"=w208, "VISA resource in"=w213, "Port to fire"=w217, "TTL pulse length, s"=w210) -> ("error out"=w214:errorcluster)  [unwired: 5 in, 2 out]
        n149 = property on="O3 Dispence, µl" class="Bool (strict)"(error in=w214, "DisabledEnum"=T1."Enabled" ("Disabled"), "Value"=w209) -> ()  [unwired: 1 in, 2 out]
      }
      event "O3 volume to dispense, µl": Value Change {
        n150 = event-data() -> ()  [unwired: 1 in, 6 out]
        n151 = property on="O3 speed, µl/s" class="DigNum (strict)"() -> ("Value"=w218:dbl)  [unwired: 2 in, 2 out]
        n152 = property on="O3 volume to dispense, µl" class="DigNum (strict)"() -> ("Value"=w220:dbl)  [unwired: 2 in, 2 out]
        n153 = Divide(x=w220, y=w218) -> (x/y=w219:dbl)
        n154 = property on="O3 time to dispense, s" class="DigNum (strict)"("Value"=w219) -> ()  [unwired: 2 in, 2 out]
      }
      event "O4 act. disp. time, s", "O4 volume, µl": Value Change {
        n155 = event-data() -> ()  [unwired: 1 in, 6 out]
        n156 = property on="O4 act. disp. time, s" class="DigNum (strict)"() -> ("Value"=w227:dbl)  [unwired: 2 in, 2 out]
        n157 = property on="O4 volume, µl" class="DigNum (strict)"() -> ("Value"=w228:dbl)  [unwired: 2 in, 2 out]
        n158 = Divide(x=w228, y=w227) -> (x/y=w222:dbl)
        n159 = property on="O4 speed, µl/s" class="DigNum (strict)"("Value"=w222) -> (error out=w225:errorcluster)  [unwired: 2 in, 1 out]
        n160 = property on="O4 Dispence, µl" class="Bool (strict)"(error in=w225, "DisabledEnum"=T1."Enabled" ("Disabled")) -> (error out=w221:errorcluster)  [unwired: 1 in, 1 out]
        n161 = property on="O4 volume to dispense, µl" class="DigNum (strict)"(error in=w221) -> ("Value"=w224:dbl)  [unwired: 1 in, 2 out]
        n162 = Divide(x=w224, y=w222) -> (x/y=w223:dbl)
        n163 = property on="O4 time to dispense, s" class="DigNum (strict)"("Value"=w223) -> ()  [unwired: 2 in, 2 out]
      }
      event "O4 Disp. by time": Value Change {
        w238 = u16 8 items=["Out 1"=1, "Out 2"=2, "Out 3"=4, "Out 4"=8] ("Port to fire")
        n164 = event-data() -> ("OldVal"=w231:bool)  [unwired: 1 in, 5 out]
        n165 = property on="O4 Disp. by time" class="Bool (strict)"(error in=w236, "DisabledEnum"=T1."Disabled and Grayed Out" ("Disabled")) -> (error out=w237:errorcluster)  [unwired: 1 in, 1 out]
        n166 = property on="O4 disp. time, s" class="DigNum (strict)"(error in=w237) -> (error out=w235:errorcluster, "Value"=w240:dbl)  [unwired: 1 in, 1 out]
        n167 = call "SW_Fire_TTL_during_calibration.vi"("error in (no error)"=w235, "VISA resource in"=w241, "Port to fire"=w238, "TTL pulse length, s"=w240) -> ("error out"=w232:errorcluster, "Time spent to process command, s"=w239:dbl)  [unwired: 5 in, 1 out]
        n168 = property on="O4 act. disp. time, s" class="DigNum (strict)"("Val(Sgnl)"=w239) -> ()  [unwired: 2 in, 2 out]
        n169 = property on="O4 Disp. by time" class="Bool (strict)"(error in=w232, "DisabledEnum"=T1."Enabled" ("Disabled"), "Value"=w231) -> (error out=w229:errorcluster)  [unwired: 1 in, 1 out]
        n170 = property on="O4 volume, µl" class="DigNum (strict)"(error in=w229, "DisabledEnum"=T1."Enabled" ("Disabled")) -> ()  [unwired: 1 in, 2 out]
      }
      event "O4 Dispence, s": Value Change {
        w249 = u16 8 items=["Out 1"=1, "Out 2"=2, "Out 3"=4, "Out 4"=8] ("Port to fire")
        n171 = event-data() -> ("OldVal"=w242:bool)  [unwired: 1 in, 5 out]
        n172 = property on="O4 Dispence, s" class="Bool (strict)"("DisabledEnum"=T1."Disabled and Grayed Out" ("Disabled")) -> (error out=w248:errorcluster)  [unwired: 2 in, 1 out]
        n173 = property on="O4 time to dispense, s" class="DigNum (strict)"(error in=w248) -> (error out=w247:errorcluster, "Value"=w250:dbl)  [unwired: 1 in, 1 out]
        n174 = call "SW_Fire_TTL_during_calibration.vi"("error in (no error)"=w247, "VISA resource in"=w243, "Port to fire"=w249, "TTL pulse length, s"=w250) -> ("error out"=w244:errorcluster)  [unwired: 5 in, 2 out]
        n175 = property on="O4 Dispence, s" class="Bool (strict)"(error in=w244, "DisabledEnum"=T1."Enabled" ("Disabled"), "Value"=w242) -> ()  [unwired: 1 in, 2 out]
      }
      event "O4 Dispence, µl": Value Change {
        w260 = u16 8 items=["Out 1"=1, "Out 2"=2, "Out 3"=4, "Out 4"=8] ("Port to fire")
        n176 = event-data() -> ("OldVal"=w252:bool)  [unwired: 1 in, 5 out]
        n177 = property on="O4 Dispence, µl" class="Bool (strict)"("DisabledEnum"=T1."Disabled and Grayed Out" ("Disabled")) -> (error out=w251:errorcluster)  [unwired: 2 in, 1 out]
        n178 = property on="O4 volume to dispense, µl" class="DigNum (strict)"() -> ("Value"=w254:dbl)  [unwired: 2 in, 2 out]
        n179 = property on="O4 speed, µl/s" class="DigNum (strict)"() -> ("Value"=w255:dbl)  [unwired: 2 in, 2 out]
        n180 = Divide(x=w254, y=w255) -> (x/y=w253:dbl)
        n181 = call "SW_Fire_TTL_during_calibration.vi"("error in (no error)"=w251, "VISA resource in"=w256, "Port to fire"=w260, "TTL pulse length, s"=w253) -> ("error out"=w257:errorcluster)  [unwired: 5 in, 2 out]
        n182 = property on="O4 Dispence, µl" class="Bool (strict)"(error in=w257, "DisabledEnum"=T1."Enabled" ("Disabled"), "Value"=w252) -> ()  [unwired: 1 in, 2 out]
      }
      event "O4 volume to dispense, µl": Value Change {
        n183 = event-data() -> ()  [unwired: 1 in, 6 out]
        n184 = property on="O4 speed, µl/s" class="DigNum (strict)"() -> ("Value"=w261:dbl)  [unwired: 2 in, 2 out]
        n185 = property on="O4 volume to dispense, µl" class="DigNum (strict)"() -> ("Value"=w263:dbl)  [unwired: 2 in, 2 out]
        n186 = Divide(x=w263, y=w261) -> (x/y=w262:dbl)
        n187 = property on="O4 time to dispense, s" class="DigNum (strict)"("Value"=w262) -> ()  [unwired: 2 in, 2 out]
      }
      event Panel Close? {
        n188 = event-data() -> ()  [unwired: 1 in, 4 out]
        n189 = event-data() -> ()  [unwired: 2 in, 1 out]
      }
      event Timeout {
        n190 = event-data() -> ()  [unwired: 1 in, 3 out]
      }
    }
  }
  n191 = while {
    tunnel: [w267] -> w1
    stop <- w266 stop-if-true
    # "This loop only for panel close purpose"
    n192 = event shown="[1] Panel Close?" {
      selector: _ -> [_ _]
      dyn-events: _ -> [_ _]
      timeout: 511 -> [_ _]
      tunnel: [_ w270] -> w267
      tunnel: [_ TRUE] -> w266
      event Timeout {
        n193 = event-data() -> ()  [unwired: 1 in, 3 out]
      }
      event Panel Close? {
        w271 = T4 128 items=["Flush Receive Buffer"=16, "Write Transmit Buffer to Device"=32, "Flush Receive Buffer (No I/O)"=64, "Flush Transmit Buffer"=128] ("Mask")
        n194 = event-data() -> ()  [unwired: 1 in, 4 out]
        n195 = property on="VISA resource" class="VISAName"() -> (error out=w280:errorcluster, "Value"=w281:refnum<visa-resource-name>)  [unwired: 2 in, 1 out]
        n196 = VISA Flush I/O Buffer(VISA resource name=w281, mask (16)=w271, error in (no error)=w280) -> (VISA resource name out=w279:refnum<visa-resource-name>, error out=w278:errorcluster)
        n197 = VISA Clear(VISA resource name=w279, error in (no error)=w278) -> (VISA resource name out=w276:refnum<visa-resource-name>, error out=w277:errorcluster)
        n198 = VISA Close(VISA resource name=w276, error in (no error)=w277) -> (error out=w275:errorcluster)
        n199 = call <vilib>:"Clear Errors.vi"("error in (no error)"=w275) -> ("error out"=w282:errorcluster)  [unwired: 5 in, 1 out]
        n200 = Current VI's Path() -> (path=w274:path)
        n201 = Open VI Reference(vi path=w274, error in (no error)=w282) -> (vi reference=w273:refnum<vi>, error out=w272:errorcluster)  [unwired: 4 in]
        n202 = invoke class="VI" method="FP.Close"(reference=w273, error in=w272) -> (error out=w270:errorcluster)  [unwired: 1 in, 2 out]
        n203 = event-data() -> ()  [unwired: 2 in, 1 out]
      }
    }
  }
  "error out" <- w1
